vi "GetSCPIVersion.vi"(8 "Fehler (Eingang, kein Fehler)":errorcluster caption="Error_In", 11 "OXYGEN Ref In":refnum<visa-resource-name>) -> (0 "Fehler (Ausgang)":errorcluster caption="Error_Out", 1 "communication_data":T1, 2 "SCPI Version":string, 3 "OXYGEN Ref Out":refnum<visa-resource-name>)   [LabVIEW 2018, in "OXYGEN.lvlib"]
doc: "Queries the implemented SCPI Standard Version."
uses:
  OXYGEN.lvlib
  TypeDefs/Cluster_RawCommData.ctl
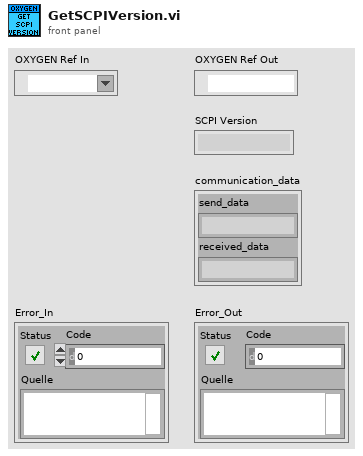
[diagram p1: front panel]
types:
  T1 = typedef "OXYGEN.lvlib/Cluster_RawCommData.ctl" = cluster{"send_data":string, "received_data":string}
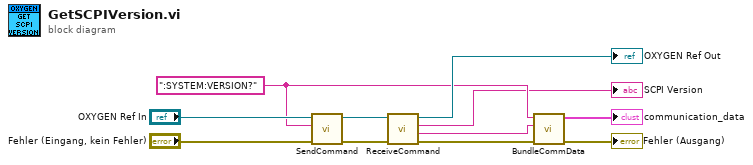
[diagram p0: block diagram]
diagram:
  w6 = ":SYSTEM:VERSION?" ("Schreibpuffer")
  n1 = call "SendCommand.vi"("error in (no error)"="Fehler (Eingang, kein Fehler)", "String to Send"=w6, "OXY_SCPI Reseource In"="OXYGEN Ref In") -> ("error out"=w8:errorcluster, "OXY_SCPI Reseource Out"=w7:refnum<visa-resource-name>)  [unwired: 7 in]
  n2 = call "ReceiveCommand.vi"("error in (no error)"=w8, "OXY_SCPI Reseource In"=w7) -> ("error out"=w4:errorcluster, "received Data with Header"=w2:string, "received Data"=→"SCPI Version":string, "OXY_SCPI Reseource Out"=→"OXYGEN Ref Out":refnum<visa-resource-name>)  [unwired: 6 in]
  n3 = call "BundleCommData.vi"("error in (no error)"=w4, "received_data"=w2, "send_data"=w6) -> ("error out"=→"Fehler (Ausgang)":errorcluster, "communication_data"=→"communication_data":T1)  [unwired: 7 in]
